vi "Get Lowest Target.vi"(1 "Target Info":T2(array[cluster])) -> (0 "Lowest Target Info":T1)   [LabVIEW 2012]
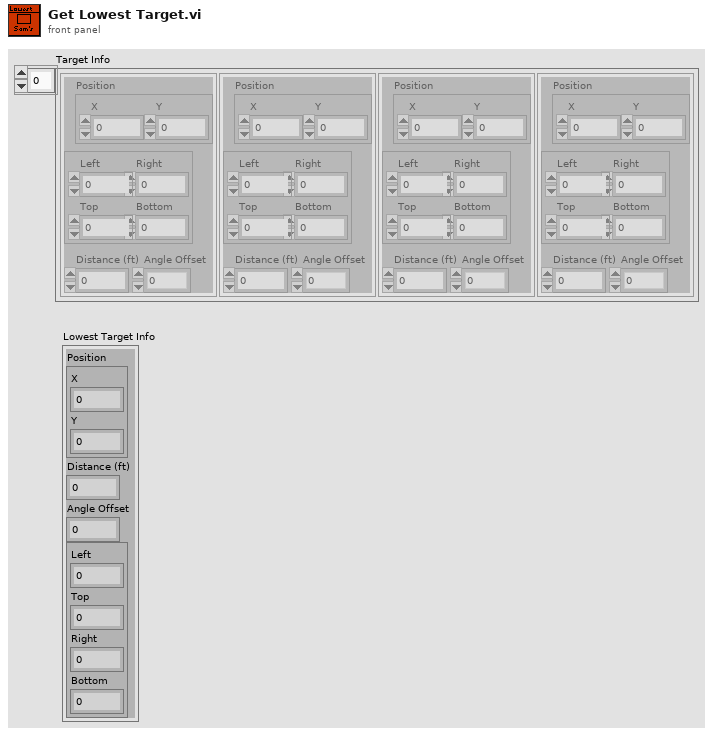
[diagram p1: front panel]
types:
  T1 = cluster{"Position":cluster{"X":dbl, "Y":dbl}, "Distance (ft)":dbl, "Angle Offset":dbl, "Bounding Box":cluster{"Left":dbl, "Top":dbl, "Right":dbl, "Bottom":dbl}}
  T2 = cluster{"Position":cluster{"X":dbl, "Y":dbl}, "Distance (ft)":dbl, "Angle Offset":dbl, "Bounding Box":cluster{"Left":dbl, "Top":dbl, "Right":dbl, "Bottom":dbl}}[]
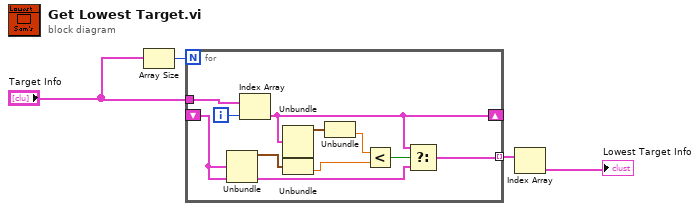
[diagram p0: block diagram]
diagram:
  n1 = Array Size(array="Target Info") -> (size(s)=w3:i32)
  n2 = for {
    N: w3 -> [_]
    tunnel: "Target Info" -> [w14]
    tunnel: [w10] -> w4 mode=indexing
    shift-right: [w8] -> _
    shift-left: _ -> [w7]
    i -> [w13]
    n3 = Unbundle(w7) -> ("Position"=w9:cluster{"X":dbl, "Y":dbl})  [unwired: 3 out]
    n4 = Index Array(array=w14, index=w13) -> (element=w8:T1)
    n5 = Unbundle(w8) -> ("Position"=w12:cluster{"X":dbl, "Y":dbl})  [unwired: 3 out]
    n6 = Unbundle(w9) -> ("Y"=w5:dbl)  [unwired: 1 out]
    n7 = Unbundle(w12) -> ("Y"=w6:dbl)  [unwired: 1 out]
    n8 = Less?(x=w6, y=w5) -> (x < y?=w11:bool)
    n9 = Select(t=w8, s=w11, f=w7) -> (s? t:f=w10:T1)
  }
  n10 = Index Array(array=w4) -> (element=→"Lowest Target Info":T1)  [unwired: 1 in]
